vi "runtime&samplecircle.vi"() -> ()   [LabVIEW 2014]
panel:
  out "Runtime":dbl
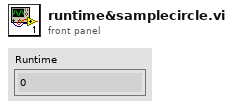
[diagram p1: front panel]
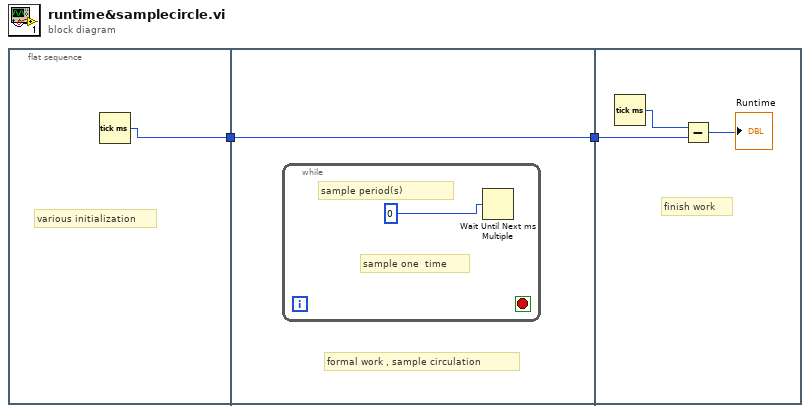
[diagram p0: block diagram]
diagram:
  n1 = flat-sequence {
    tunnel: [w3] -> w1
    tunnel: [w4] -> w2
    tunnel: w1 -> [w4]
    tunnel: w2 -> [w6]
    frame #0 {
      # "various initialization"
      n2 = Tick Count (ms)() -> (millisecond timer value=w3:u32)
    }
    frame #1 {
      # "formal work , sample circulation"
      n3 = while {
        stop <- _ stop-if-true
        # "sample one  time"
        # "sample period(s)"
        n4 = Wait Until Next ms Multiple(millisecond multiple=0) -> ()  [unwired: 1 out]
      }
    }
    frame #2 {
      # "finish work"
      n5 = Tick Count (ms)() -> (millisecond timer value=w7:u32)
      n6 = Subtract(x=w7, y=w6) -> (x-y=→"Runtime":u32)
    }
  }
